vi "Read Profiles from Target.vi"(8 "error in (no error)":errorcluster, 9 "directory path":string, 10 "protocol":T4=enum."WebDAV", 11 "session in":T1) -> (0 "error out":errorcluster, 2 "Fies":string[](array[string]), 3 "session out":T1)   [LabVIEW 2019, in "Scan Engine Custom Device.lvlib"]
uses:
  Scan Engine Custom Device.lvlib
  <resource>/Framework/Providers/indcomecat/_InternalSubVIs/_fileTransferProtocol.ctl
  <resource>/Framework/Providers/indcomecat/_InternalSubVIs/_protocolSession.ctl
  <vilib>/FTP/ftp0.llb/FTP Session.ctl
  <vilib>/WebDAVClient/Advanced/SessionHandle.ctl
  <vilib>/FTP/NI_FTP.lvlib
  <vilib>/WebDAVClient/NI_WebDAV.lvlib
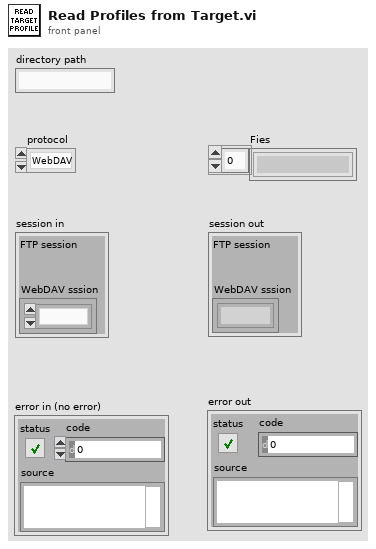
[diagram p1: front panel]
types:
  T1 = typedef "_protocolSession.ctl" = cluster{"FTP session":T2, "WebDAV sssion":T3}
  T2 = typedef "NI_FTP.lvlib/FTP Session.ctl" = refnum<k5>
  T3 = typedef "NI_WebDAV.lvlib/SessionHandle.ctl" = refnum<k1>
  T4 = typedef "_fileTransferProtocol.ctl" = enum16{"Ftp", "WebDAV", "None"}
  T5 = typedef "NI_FTP.lvlib/FTP File Info.ctl" = cluster{"type":enum16{"unknown", "file", "dir", "link"}, "permissions":string, "owner":string, "group":string, "size":i32, "date":string, "name":string, "link name":string}
  T6 = typedef "NI_WebDAV.lvlib/FileInfo.ctl" = cluster{"type":string, "size":u64, "last modification":timestamp, "display name":string, "uri":string}
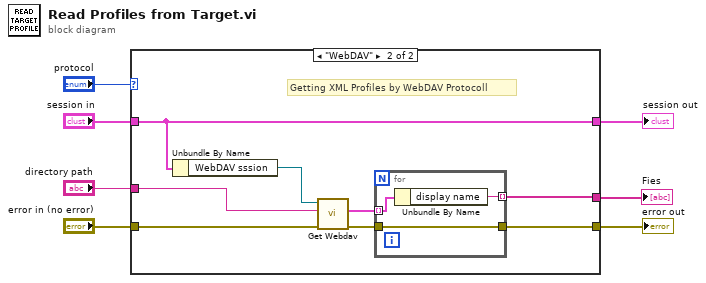
[diagram p0: block diagram]
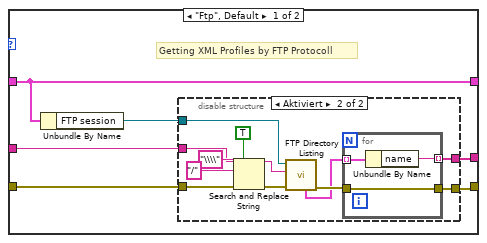
[diagram p2: hidden frame]
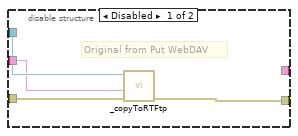
[diagram p3: hidden frame]
diagram:
  n1 = case shown="\"WebDAV\"" "protocol" {
    tunnel: "session in" -> [w11 w38]
    tunnel: [w10 w35] -> w3
    tunnel: "error in (no error)" -> [w13 w39]
    tunnel: [w11 w38] -> w4
    tunnel: "directory path" -> [w9 w37]
    tunnel: [w8 w33] -> w1
    frame "Ftp", Default {
      # "Getting XML Profiles by FTP Protocoll"
      n2 = Unbundle By Name(w11) -> ("FTP session"=w12:T2)
      n3 = disable-structure shown="Aktiviert" {
        disable-tunnel: w13 -> [w17 w26]
        disable-tunnel: w12 -> [w16 w24]
        disable-tunnel: [w15 w21] -> w10
        disable-tunnel: w9 -> [w14 w27]
        disable-tunnel: [_ w20] -> w8
        frame Disabled {
          # "Original from Put WebDAV"
          n4 = call <resource>:"_copyToRTFtp.vi"("error in (no error)"=w17, "directory path"=w14, "TCP Network Connection in"=w16) -> ("error out"=w15:errorcluster)  [unwired: 7 in, 1 out]
        }
        frame Enabled {
          n5 = Search and Replace String(replace all?=TRUE ("replace all? (F)"), input string=w27, search string="\\\\", replace string="/" ("replace string (\"\")"), error in=w26) -> (result string=w23:string, error out=w25:errorcluster)  [unwired: 3 in, 2 out]
          n6 = call <vilib>:"FTP Directory Listing.vi"("error in (no error)"=w25, "directory path"=w23, "ftp session"=w24) -> ("error out"=w22:errorcluster, "dir list"=w19:T5[])  [unwired: 4 in, 3 out]
          n7 = for {
            tunnel: w22 -> [w32]
            tunnel: [w32] -> w21
            tunnel: w19 -> [w31] mode=indexing
            tunnel: [w30] -> w20 mode=indexing
            n8 = Unbundle By Name(w31) -> ("name"=w30:string)
          }
        }
      }
    }
    frame "WebDAV" {
      # "Getting XML Profiles by WebDAV Protocoll"
      n9 = Unbundle By Name(w38) -> ("WebDAV sssion"=w40:T3)
      n10 = call "Get Webdav.vi"("error in (no error)"=w39, "relative uri"=w37, "Refnum in"=w40) -> ("error out"=w36:errorcluster, "file list"=w34:T6[])  [unwired: 6 in, 1 out]
      n11 = for {
        tunnel: w36 -> [w43]
        tunnel: [w43] -> w35
        tunnel: w34 -> [w42] mode=indexing
        tunnel: [w41] -> w33 mode=indexing
        n12 = Unbundle By Name(w42) -> ("display name"=w41:string)
      }
    }
  }
  "error out" <- w3
  "session out" <- w4
  "Fies" <- w1
